vi "test Get-Set Logging Properties.vi"(8 "error in":errorcluster, 11 "TestCase in":refnum<class "Scripting.lvclass">) -> (0 "error out":errorcluster, 3 "TestCase out":refnum<class "Scripting.lvclass">)   [LabVIEW 2020, in "Scripting.lvclass"]
uses:
  Scripting.lvclass
  Scripting/AIM MIL-STD-1553 Scripting.lvlib
  <vilib>/addons/_JKI Toolkits/VI Tester/TestCase.llb/TestCase.lvclass
  Shared/Data Word Format.ctl
  C:/dev/git/niveristand-custom-device-testing-tools/VeriStandScriptingTestCase/VeriStandScriptingTestCase.lvclass
  C:/Program Files (x86)/National Instruments/LabVIEW 2020/vi.lib/addons/_JKI Toolkits/VI Tester/TestCase.llb/TestCase.lvclass
  C:/dev/git/niveristand-aim-milStd1553-custom-device/Source/Custom Device Support/Tests/Unit/Scripting/Scripting.lvclass
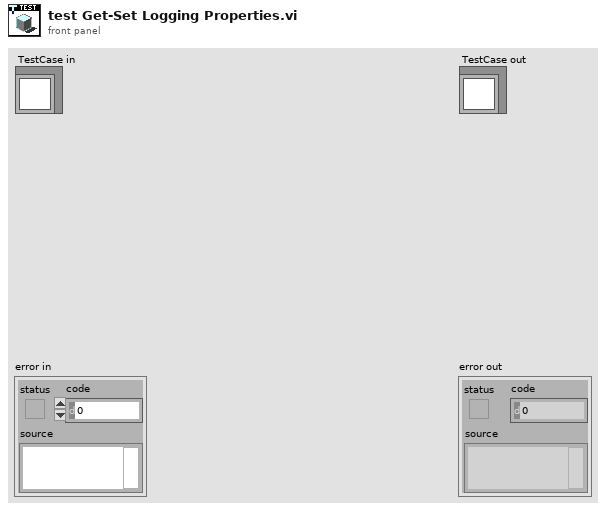
[diagram p1: front panel]
types:
  T1 = typedef "Data Word Format.ctl" = string
  T2 = typedef "Custom Device API.lvlib/Custom Device Item Ref.ctl" = u64
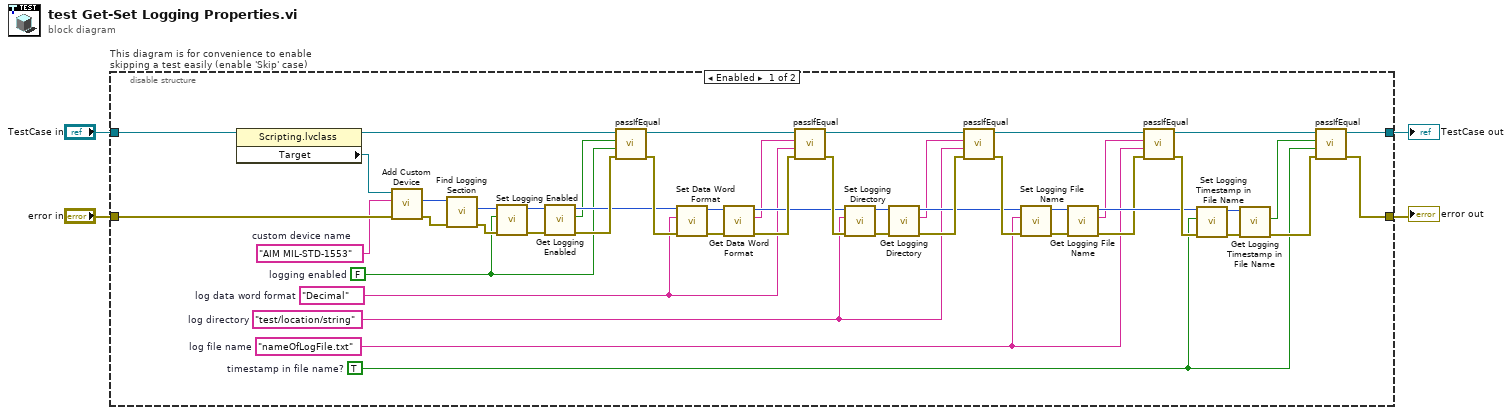
[diagram p0: block diagram]
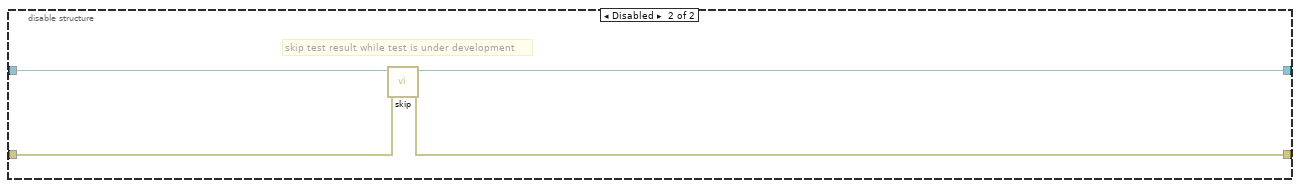
[diagram p2: hidden frame]
diagram:
  n1 = disable-structure "This diagram is for convenience to enable skipping a test easily (enable 'Skip' case)" shown="Enabled" {
    disable-tunnel: "TestCase in" -> [w48 w56]
    disable-tunnel: [w50 w54] -> w4
    disable-tunnel: [w49 w55] -> w2
    disable-tunnel: "error in" -> [w52 w53]
    frame Enabled {
      w5 = TRUE  # timestamp in file name?
      w6 = "nameOfLogFile.txt"  # log file name
      w7 = "test/location/string"  # log directory
      w8 = T1 "Decimal"  # log data word format
      w9 = FALSE  # logging enabled
      w51 = "AIM MIL-STD-1553"  # custom device name
      n2 = property class="Scripting.lvclass"(reference=w48) -> (reference out=w34:refnum<class "Scripting.lvclass">, "Target"=w47:refnum<k24>)  [unwired: 1 in, 1 out]
      n3 = call "Add Custom Device.vi"("error in"=w52, "custom device name"=w51, "target"=w47) -> ("error out"=w45:errorcluster, "custom device"=w46:T2)  [unwired: 6 in, 1 out]
      n4 = call "Find Logging Section.vi"("error in"=w45, "custom device"=w46) -> ("error out"=w43:errorcluster, "logging section"=w44:T2)  [unwired: 7 in, 1 out]
      n5 = call "Set Logging Enabled.vi"("error in"=w43, "logging enabled"=w9, "logging section"=w44) -> ("error out"=w42:errorcluster, "logging section out"=w41:T2)  [unwired: 7 in]
      n6 = call "Get Logging Enabled.vi"("error in"=w42, "logging section"=w41) -> ("error out"=w40:errorcluster, "logging enabled"=w14:bool, "logging section out"=w24:T2)  [unwired: 7 in]
      n7 = call-dynamic "passIfEqual.vi"("error in (no error)"=w40, "y"=w9, "x"=w14, "TestCase in"=w34) -> ("error out"=w39:errorcluster, "TestCase out"=w33:refnum<class "Scripting.lvclass">)  [unwired: 6 in]
      n8 = call "Set Data Word Format.vi"("error in"=w39, "data word format"=w8, "logging section"=w24) -> ("error out"=w38:errorcluster, "logging section out"=w37:T2)  [unwired: 7 in]
      n9 = call "Get Data Word Format.vi"("error in"=w38, "logging section"=w37) -> ("error out"=w36:errorcluster, "data word format"=w13:T1, "logging section out"=w25:T2)  [unwired: 7 in]
      n10 = call-dynamic "passIfEqual.vi"("error in (no error)"=w36, "y"=w8, "x"=w13, "TestCase in"=w33) -> ("error out"=w35:errorcluster, "TestCase out"=w32:refnum<class "Scripting.lvclass">)  [unwired: 6 in]
      n11 = call "Set Logging Directory.vi"("error in"=w35, "directory"=w7, "logging section"=w25) -> ("error out"=w27:errorcluster, "logging section out"=w26:T2)  [unwired: 6 in]
      n12 = call "Get Logging Directory.vi"("error in"=w27, "logging section"=w26) -> ("error out"=w23:errorcluster, "directory"=w12:string, "logging section out"=w19:T2)  [unwired: 7 in]
      n13 = call-dynamic "passIfEqual.vi"("error in (no error)"=w23, "y"=w7, "x"=w12, "TestCase in"=w32) -> ("error out"=w29:errorcluster, "TestCase out"=w31:refnum<class "Scripting.lvclass">)  [unwired: 6 in]
      n14 = call "Set Logging File Name.vi"("error in"=w29, "file name"=w6, "logging section"=w19) -> ("error out"=w22:errorcluster, "logging section out"=w18:T2)  [unwired: 6 in]
      n15 = call "Get Logging File Name.vi"("error in"=w22, "logging section"=w18) -> ("error out"=w16:errorcluster, "file name"=w11:string, "logging section out"=w17:T2)  [unwired: 7 in]
      n16 = call-dynamic "passIfEqual.vi"("error in (no error)"=w16, "y"=w6, "x"=w11, "TestCase in"=w31) -> ("error out"=w28:errorcluster, "TestCase out"=w30:refnum<class "Scripting.lvclass">)  [unwired: 6 in]
      n17 = call "Set Logging Timestamp in File Name.vi"("error in"=w28, "timestamp in file name"=w5, "logging section"=w17) -> ("error out"=w20:errorcluster, "logging section out"=w21:T2)  [unwired: 7 in]
      n18 = call "Get Logging Timestamp in File Name.vi"("error in"=w20, "logging section"=w21) -> ("error out"=w15:errorcluster, "timestamp in file name"=w10:bool)  [unwired: 7 in, 1 out]
      n19 = call-dynamic "passIfEqual.vi"("error in (no error)"=w15, "y"=w5, "x"=w10, "TestCase in"=w30) -> ("error out"=w49:errorcluster, "TestCase out"=w50:refnum<class "Scripting.lvclass">)  [unwired: 6 in]
    }
    frame Disabled {
      # "skip test result while test is under development"
      n20 = call <vilib>:"skip.vi"("error in (no error)"=w53, "TestCase in"=w56) -> ("error out"=w55:errorcluster, "TestCase out"=w54:refnum<class "Scripting.lvclass">)  [unwired: 8 in]
    }
  }
  "error out" <- w2
  "TestCase out" <- w4
